vi "initiate.vi"(0 "reference in":refnum<class "excelFile.lvclass">, 5 "error in (no error)":errorcluster) -> (14 "reference out":refnum<class "excelFile.lvclass">, 19 "error out":errorcluster)   [LabVIEW 2015, in "excelFile.lvclass"]
uses:
  excelFile.lvclass
  python_class/python.lvclass
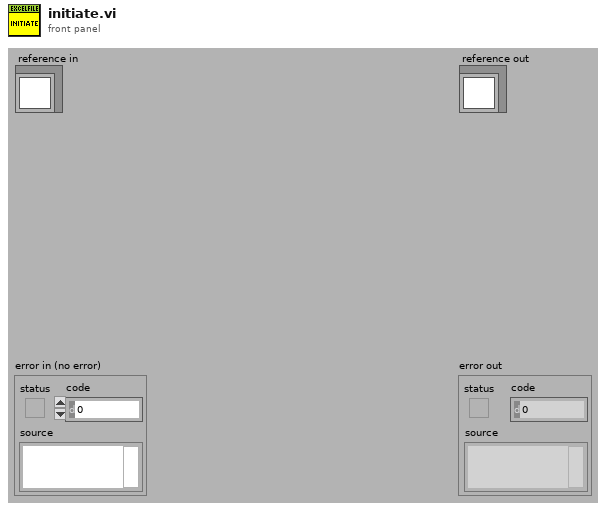
[diagram p1: front panel]
types:
  T1 = typedef "excelFile.lvclass/ObjectAttributesRef.ctl" = refnum<data-value>
  T2 = typedef "excelFile.lvclass/ObjectAttributes.ctl" = cluster{"MyAttribute":dbl, "path":string, "Refnum Excel":cluster{"Excel._Application":refnum<k7>, "Workbooks":refnum<k7>, "Open":refnum<k7>}, "data":string[][][], "save":bool, "fileType":T3, "rowsColor":u32[], "python_ref":refnum<class "python.lvclass">, "items_rows":i32[], "excel_range":i32[][], "TSR":cluster{"number":string, "TSR_path":path, "service_path":path, "email_to":string}, "excel_already_opened?":bool, "file_already_opened?":bool, "excel_protected_opened?":bool}
  T3 = typedef "excelFile.lvclass/fileType.ctl" = enum16{"devices", "items", "partsTracking", "TSR"}
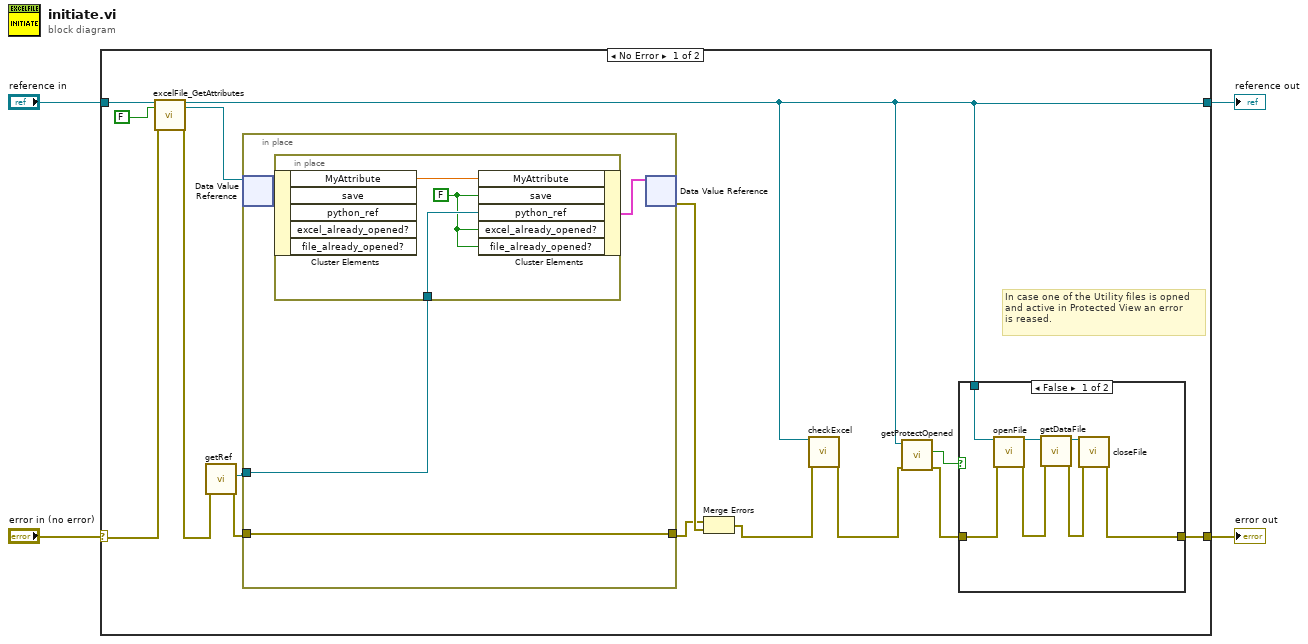
[diagram p0: block diagram]
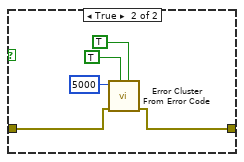
[diagram p2: hidden frame]
diagram:
  n1 = case shown="No Error" "error in (no error)" {
    selector: "error in (no error)" -> [w15 w40]
    tunnel: [w10 w40] -> w3
    tunnel: [w8 w39] -> w1
    tunnel: "reference in" -> [w17 w39]
    frame No Error {
      # "In case one of the Utility files is opned\nand active in Protected View an error\nis reased."
      n2 = call "excelFile_GetAttributes.vi"("reference in"=w17, "return data? (T)"=FALSE, "error in (no error)"=w15) -> ("reference out"=w8:refnum<class "excelFile.lvclass">, "attributes ref"=w14:T1, "error out"=w13:errorcluster)  [unwired: 13 in, 1 out]
      n3 = call "getRef.vi"("error in (no error)"=w13) -> ("error out"=w12:errorcluster, "python_ref"=w11:refnum<class "python.lvclass">)  [unwired: 9 in]
      n4 = in-place {
        in-place-border: w12 -> [w33]
        in-place-border: [w33] -> w18
        in-place-border: w11 -> [w32]
        n5 = in-place-dvr #1(w14) -> (w34:T2)  [unwired: 1 out]
        n6 = in-place {
          in-place-border: w32 -> [w37]
          w36 = FALSE ("save")
          n7 = in-place-cluster #2(w34) -> ("MyAttribute"=w38:dbl)  [unwired: 4 out]
          n8 = in-place-cluster #2("MyAttribute"=w38, "save"=w36, "python_ref"=w37, "excel_already_opened?"=w36, "file_already_opened?"=w36) -> (w35:T2)
        }
        n9 = in-place-dvr #1(w35) -> (w19:errorcluster)  [unwired: 1 out]
      }
      n10 = Merge Errors(w18, w19) -> (w9:errorcluster)
      n11 = call "checkExcel.vi"("reference in"=w8, "error in (no error)"=w9) -> ("error out"=w7:errorcluster)  [unwired: 16 in, 1 out]
      n12 = call "getProtectOpened.vi"("error in (no error)"=w7, "reference in"=w8) -> ("error out"=w6:errorcluster, "excel_protected_opened?"=w5:bool)  [unwired: 7 in, 1 out]
      n13 = case shown="False" w5 {
        tunnel: [w24 w30] -> w10
        tunnel: w8 -> [w20 _]
        tunnel: w6 -> [w21 w31]
        frame False {
          n14 = call "openFile.vi"("reference in"=w20, "error in (no error)"=w21) -> ("reference out"=w23:refnum<class "excelFile.lvclass">, "error out"=w26:errorcluster)  [unwired: 16 in]
          n15 = call "getDataFile.vi"("error in (no error)"=w26, "reference in"=w23) -> ("error out"=w25:errorcluster, "reference out"=w22:refnum<class "excelFile.lvclass">)  [unwired: 8 in]
          n16 = call "closeFile.vi"("error in (no error)"=w25, "reference in"=w22) -> ("error out"=w24:errorcluster)  [unwired: 8 in, 1 out]
        }
        frame True {
          n17 = call <vilib>:"Error Cluster From Error Code.vi"("is warning? (False)"=TRUE, "show call chain? (False)"=TRUE, "error in (no error)"=w31, "error code (0)"=5000 ("error code (no error:0)")) -> ("error out"=w30:errorcluster)  [unwired: 5 in]
        }
      }
    }
    frame Error {
    }
  }
  "error out" <- w3
  "reference out" <- w1
